vi "AddFailure.vi"(7 "Time":dbl, 8 "error in (no error)":errorcluster, 9 "Failure":errorcluster, 10 "Test":refnum<class "Test.lvclass">, 11 "FakeTestListener in":refnum<class "FakeTestListener.lvclass">) -> (0 "error out":errorcluster, 3 "FakeTestListener out":refnum<class "FakeTestListener.lvclass">)   [LabVIEW 2019, in "TestResultTest.lvlib" / "Support.lvlib" / "FakeTestListener.lvclass"]
doc: "A failure occurred."
uses:
  FakeTestListener.lvclass
  Test/Test.lvclass
  FakeTestListener.lvclass/FakeTestListener.ctl
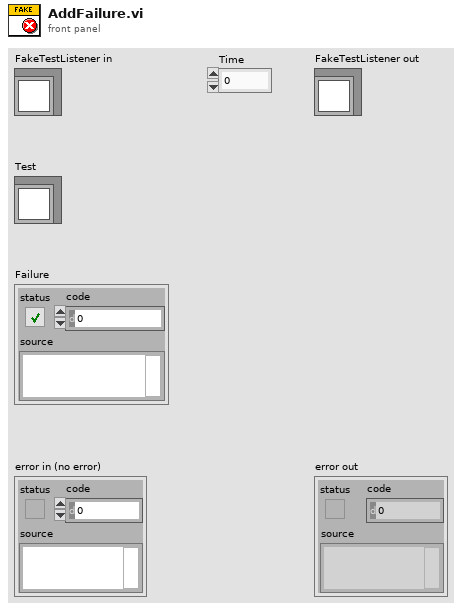
[diagram p1: front panel]
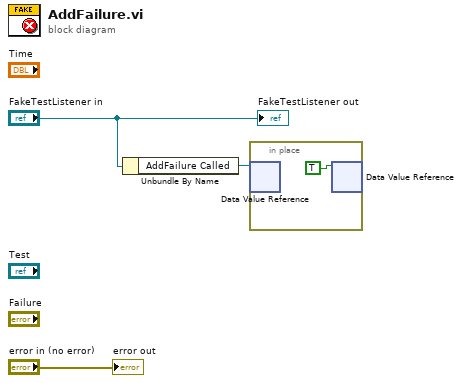
[diagram p0: block diagram]
diagram:
  n1 = Unbundle By Name("FakeTestListener in") -> ("AddFailure Called"=w1:refnum<data-value>)
  n2 = in-place {
    n3 = in-place-dvr #1(w1) -> ()  [unwired: 2 out]
    n4 = in-place-dvr #1(TRUE ("data value")) -> ()  [unwired: 2 out]
  }
  "error out" <- "error in (no error)"
  "FakeTestListener out" <- "FakeTestListener in"
